vi "uService to launch at startup.vi"(8 "error in (no error)":errorcluster, 11 "Guardian in":refnum<class "Guardian.lvclass">) -> (0 "error out":errorcluster, 3 "Guardian out":refnum<class "Guardian.lvclass">)   [LabVIEW 2026, in "TALOS.lvlib" / "Guardian.lvlib" / "Guardian.lvclass"]
doc: "This VI reads the list of uService to be autostarted on this PC and add them to the starting queue."
uses:
  Guardian.lvclass
  C:/LabVIEW Code/TALOS/builds/Actor Framework PPL/Actor Framework.lvlibp/1abvi3w/vi.lib/ActorFramework/Actor/Actor.lvclass
  Guardian Messages/Launch uService Msg/Launch uService Msg.lvclass
  C:/LabVIEW Code/TALOS/builds/Actor Framework PPL/Actor Framework.lvlibp/1abvi3w/vi.lib/ActorFramework/Message/Message.lvclass
  Guardian Messages/Launch uService Msg/Launch uService Msg.lvclass/Launch uService Msg.ctl
  Ancestor/Ancestor/Ancestor.lvclass/Ancestor.ctl
  Support VIs/Generate Error.vi
  FGV/Error Memory/Get Error Description.vi
  Support VIs/Get PC name.vi
  Ancestor/Ancestor/Read ID.vi
  Support VIs/Get Class Name.vi
  <vilib>/Utility/error.llb/Clear Errors.vi
  FGV/Error Memory/Error Memory Core.vi
  <vilib>/AdvancedString/Delimited String to 1D String Array.vi
  <vilib>/AdvancedString/Delimited String to 1D String Array (string).vi
  Support VIs/Circus Root Path.vi
  FGV/Error Memory/Error Crt Lvl checker.vi
  FGV/Error Memory/Error Memory Core.vi/40c8088d-b597-4017-91af-faa98e00292e.vi
  FGV/Error Memory/Error Memory Core.vi/d4a3ab98-063c-4e44-b43d-fbdcfe6c2be2.vi
  Support VIs/Global Memory.vi
  <vilib>/Utility/LVClass/Get LV Class Name.vi
  Support VIs/Is in Packed Library.vi
  Support VIs/TALOS Root path.vi
  Support VIs/Read CSV worksheet.vi
  Support VIs/Global Constants.vi
  <vilib>/Utility/error.llb/General Error Handler.vi
  Support VIs/Error Log.vi
  Ancestor/Ancestor/Ancestor.lvclass
  <vilib>/Comparison/Equal/Equal Functor/Equal Functor.lvclass
  builds/Actor Framework PPL/Actor Framework.lvlibp/1abvi3w/vi.lib/ActorFramework/Actor/Actor.lvclass
  builds/Actor Framework PPL/Actor Framework.lvlibp
  TALOS.lvlib
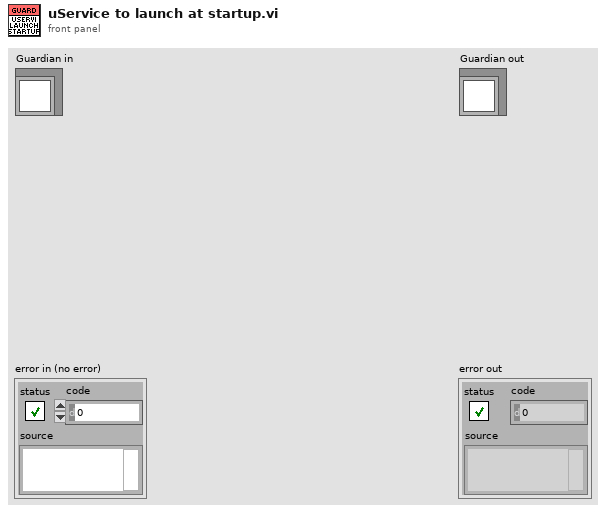
[diagram p1: front panel]
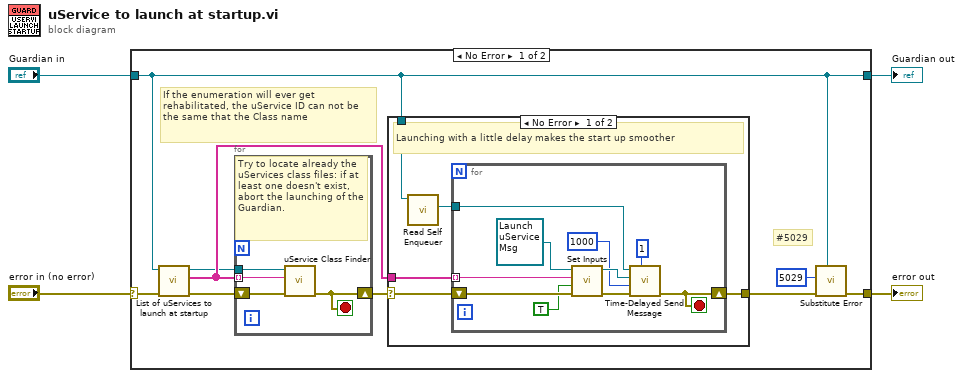
[diagram p0: block diagram]
diagram:
  n1 = case shown="No Error" "error in (no error)" {
    selector: "error in (no error)" -> [w13 w35]
    tunnel: [w7 w35] -> w3
    tunnel: [w5 w34] -> w1
    tunnel: "Guardian in" -> [w5 w34]
    frame No Error {
      # "#5029"
      # "If the enumeration will ever get rehabilitated, the uService ID can not be the same that the Class name"
      n2 = call "List of uServices to launch at startup.vi"("error in (no error)"=w13, "Guardian in"=w5) -> ("error out"=w12:errorcluster, "Array"=w10:string[], "Guardian out"=w9:refnum<class "Guardian.lvclass">)  [unwired: 7 in]
      n3 = for {
        tunnel: w10 -> [w32] mode=indexing
        shift-right: [w30] -> w11
        shift-left: w12 -> [w33]
        tunnel: w9 -> [w31]
        stop <- w30 stop-if-true
        # "Try to locate already the uServices class files: if at least one doesn't exist, abort the launching of the Guardian."
        n4 = call "uService Class Finder.vi"("error in (no error)"=w33, "uService Class name"=w32, "Guardian in"=w31) -> ("error out"=w30:errorcluster)  [unwired: 5 in, 3 out]
      }
      n5 = case shown="No Error" w11 {
        selector: w11 -> [w15 w29]
        tunnel: w10 -> [w17 _]
        tunnel: w5 -> [w16 _]
        tunnel: [w14 w29] -> w8
        frame No Error {
          # "Launching with a little delay makes the start up smoother"
          n6 = call "Read Self Enqueuer.vi"("Actor"=w16) -> ("Self Enqueuer"=w18:refnum<class "Message Enqueuer.lvclass">)  [unwired: 10 in]
          n7 = for {
            tunnel: w18 -> [w28]
            tunnel: w17 -> [w27] mode=indexing
            shift-right: [w25] -> w14
            shift-left: w15 -> [w26]
            stop <- w25 stop-if-true
            n8 = call "Set Inputs.vi"("error in (no error)"=w26, "GUI?"=TRUE, "uService Class Name"=w27, "Launch uService Msg in"=refnum<class "Launch uService Msg.lvclass"> refnum ("TALOS.lvlib:Guardian.lvlib:Launch uService Msg.lvclass")) -> ("error out"=w19:errorcluster, "Launch uService Msg out"=w22:refnum<class "Launch uService Msg.lvclass">)  [unwired: 6 in]
            n9 = call "Time-Delayed Send Message.vi"("# Copies (0 = infinite repeat)"=u32 1, "error in (no error)"=w19, "Milliseconds To Wait"=1000, "Message"=w22, "Message Enqueuer"=w28) -> ("error out"=w25:errorcluster)  [unwired: 5 in, 1 out]
          }
        }
        frame Error {
        }
      }
      n10 = call "Substitute Error.vi"("LabVIEW Object"=w5, "error in (no error)"=w8, "Error Code"=5029) -> ("error out"=w7:errorcluster)  [unwired: 8 in]
    }
    frame Error {
    }
  }
  "error out" <- w3
  "Guardian out" <- w1
